vi "Get Horizontal Speed.vi"(10 "speed":i32, 11 "index":i32) -> (2 "speed out":i32, 3 "function return":u32)   [LabVIEW 2018, in "AndorSDK.lvlib"]
doc: "EXPNETTYPE unsigned int WINAPI GetHorizontalSpeed(int index, int * speed);"
uses:
  AndorSDK.lvlib
  ATMCD32D.dll
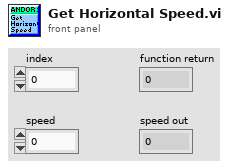
[diagram p1: front panel]
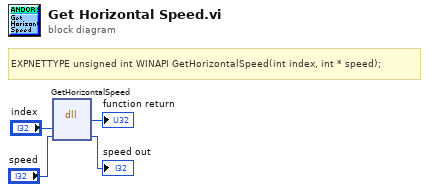
[diagram p0: block diagram]
diagram:
  # "EXPNETTYPE unsigned int WINAPI GetHorizontalSpeed(int index, int * speed);"
  n1 = dll-call lib="PTH2babs E\nPersönliches02 - Arbeit03-HiwijobsLabviewCodelibANDOR\tAndor SDK\nATMCD32D.*" fn="GetHorizontalSpeed"("index"="index", "speed"="speed") -> (→"function return":u32, "speed"=→"speed out":i32)  [unwired: 4 in, 2 out]
